vi "MSScript_SubVI_SentenceIdentifier.vi"(5 "IniPosition":i32, 6 "strlen":i32, 7 "Single sentance in":string) -> (0 "Delimiter SELs":cluster{"Start":u32, "End":u32}[](array[cluster]), 1 "Parameter string":cluster{"Str":string, "Start":i32}, 2 "Name string":cluster{"Str":string, "Start":i32}, 3 "Sentence type":string)   [LabVIEW 2018, in "MSScript.lvclass"]
uses:
  MSScript.lvclass
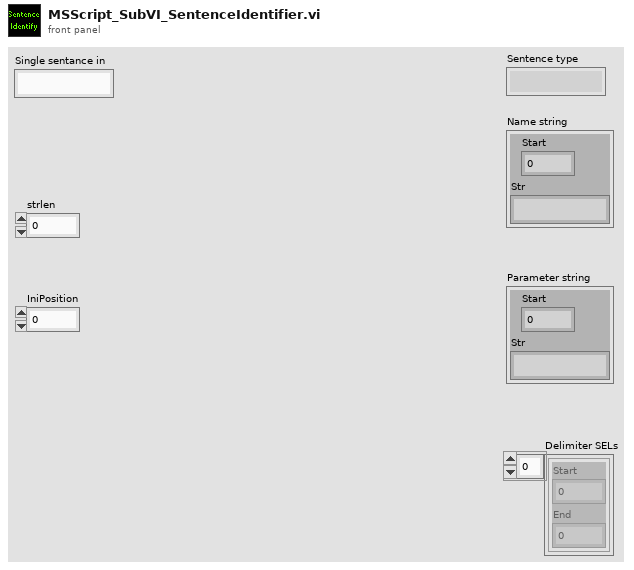
[diagram p1: front panel]
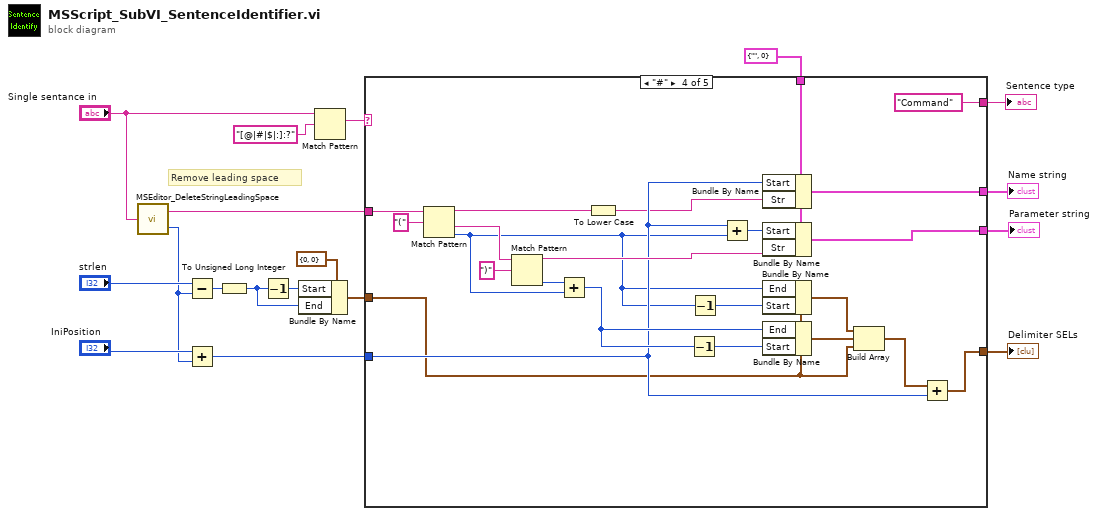
[diagram p0: block diagram]
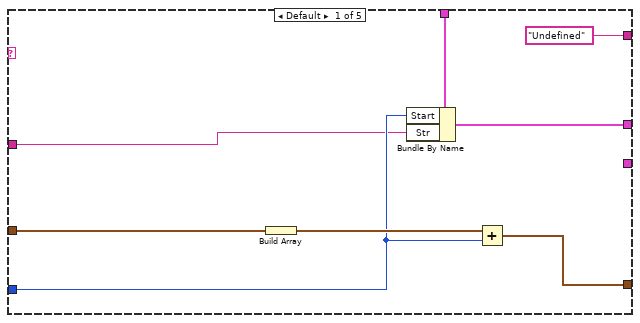
[diagram p2: hidden frame]
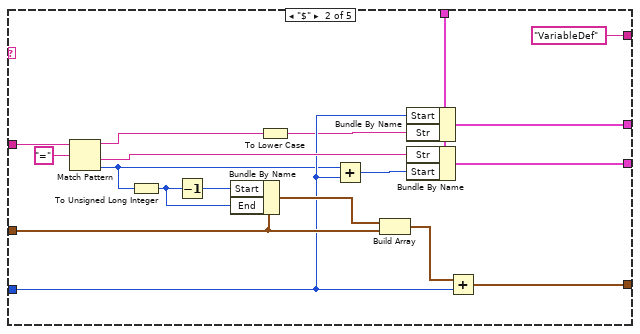
[diagram p3: hidden frame]
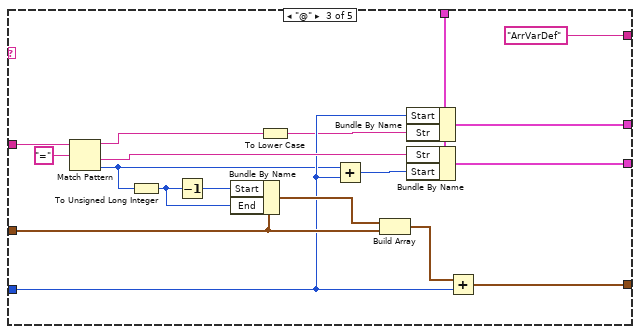
[diagram p4: hidden frame]
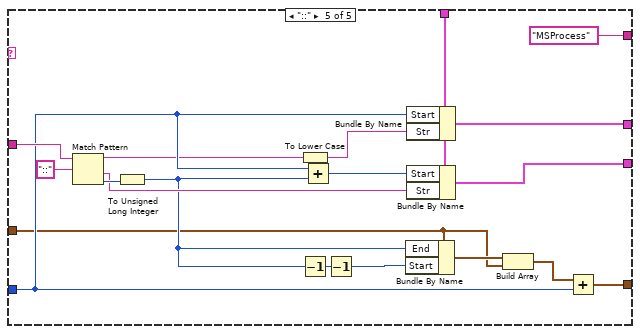
[diagram p5: hidden frame]
diagram:
  # "Remove leading space"
  n1 = call "MSEditor_DeleteStringLeadingSpace.vi"("string in"="Single sentance in") -> ("string after leading space"=w6:string, "offset past leading space"=w2:i32)
  n2 = Subtract(x="strlen", y=w2) -> (x-y=w4:i32)
  n3 = Add(x="IniPosition", y=w2) -> (x+y=w1:i32)
  n4 = To Unsigned Long Integer(number=w4) -> (unsigned 32bit integer=w10:u32)
  n5 = Decrement(x=w10) -> (x-1=w17:u32)
  n6 = Bundle By Name(cluster=cluster{"Start":u32, "End":u32} {"Start"=0, "End"=0}, "Start"=w17, "End"=w10) -> (w16:cluster{"Start":u32, "End":u32})
  n7 = Match Pattern(string="Single sentance in", regular expression="[@|#|$|:]:?") -> (match substring=w18:string)  [unwired: 1 in, 3 out]
  n8 = case shown="\"#\"" w18 {
    tunnel: w6 -> [w20 w35 w53 w81 w103]
    tunnel: ["Undefined" "VariableDef" "ArrVarDef" "Command" "MSProcess"] -> w14
    tunnel: w16 -> [w25 w38 w56 w65 w89]
    tunnel: [w23 w37 w55 w71 w95] -> w15
    tunnel: [_ w39 w57 w78 w102] -> w12
    tunnel: [w19 w29 w47 w80 w91] -> w13
    tunnel: cluster{"Str":string, "Start":i32} {"Str"="", "Start"=0} -> [w22 w30 w48 w67 w90]
    tunnel: w1 -> [w21 w33 w51 w69 w94]
    frame Default {
      n9 = Build Array(w25) -> (w24:cluster{"Start":u32, "End":u32}[])
      n10 = Bundle By Name(cluster=w22, "Start"=w21, "Str"=w20) -> (w19:cluster{"Str":string, "Start":i32})
      n11 = Add(x=w24, y=w21) -> (x+y=w23:cluster{"Start":u32, "End":u32}[])
    }
    frame "$" {
      n12 = Match Pattern(string=w35, regular expression="=") -> (before substring=w28:string, after substring=w34:string, offset past match=w32:i32)  [unwired: 1 in, 1 out]
      n13 = To Unsigned Long Integer(number=w32) -> (unsigned 32bit integer=w36:u32)
      n14 = Decrement(x=w36) -> (x-1=w42:u32)
      n15 = Bundle By Name(cluster=w38, "Start"=w42, "End"=w36) -> (w41:cluster{"Start":u32, "End":u32})
      n16 = To Lower Case(string=w28) -> (all lower case string=w27:string)
      n17 = Add(x=w32, y=w33) -> (x+y=w31:i32)
      n18 = Build Array(w41, w38) -> (w40:cluster{"Start":u32, "End":u32}[])
      n19 = Bundle By Name(cluster=w30, "Start"=w33, "Str"=w27) -> (w29:cluster{"Str":string, "Start":i32})
      n20 = Bundle By Name(cluster=w30, "Str"=w34, "Start"=w31) -> (w39:cluster{"Str":string, "Start":i32})
      n21 = Add(x=w40, y=w33) -> (x+y=w37:cluster{"Start":u32, "End":u32}[])
    }
    frame "@" {
      n22 = Match Pattern(string=w53, regular expression="=") -> (before substring=w46:string, after substring=w52:string, offset past match=w50:i32)  [unwired: 1 in, 1 out]
      n23 = To Unsigned Long Integer(number=w50) -> (unsigned 32bit integer=w54:u32)
      n24 = Decrement(x=w54) -> (x-1=w60:u32)
      n25 = Bundle By Name(cluster=w56, "Start"=w60, "End"=w54) -> (w59:cluster{"Start":u32, "End":u32})
      n26 = To Lower Case(string=w46) -> (all lower case string=w45:string)
      n27 = Add(x=w50, y=w51) -> (x+y=w49:i32)
      n28 = Build Array(w59, w56) -> (w58:cluster{"Start":u32, "End":u32}[])
      n29 = Bundle By Name(cluster=w48, "Start"=w51, "Str"=w45) -> (w47:cluster{"Str":string, "Start":i32})
      n30 = Bundle By Name(cluster=w48, "Str"=w52, "Start"=w49) -> (w57:cluster{"Str":string, "Start":i32})
      n31 = Add(x=w58, y=w51) -> (x+y=w55:cluster{"Start":u32, "End":u32}[])
    }
    frame "#" {
      n32 = Match Pattern(string=w81, regular expression="(") -> (before substring=w64:string, after substring=w82:string, offset past match=w68:i32)  [unwired: 1 in, 1 out]
      n33 = Match Pattern(string=w82, regular expression=")") -> (before substring=w79:string, offset past match=w77:i32)  [unwired: 1 in, 2 out]
      n34 = Add(x=w77, y=w68) -> (x+y=w75:i32)
      n35 = To Lower Case(string=w64) -> (all lower case string=w63:string)
      n36 = Decrement(x=w75) -> (x-1=w74:i32)
      n37 = Decrement(x=w68) -> (x-1=w76:i32)
      n38 = Add(x=w69, y=w68) -> (x+y=w70:i32)
      n39 = Bundle By Name(cluster=w67, "Start"=w69, "Str"=w63) -> (w80:cluster{"Str":string, "Start":i32})
      n40 = Bundle By Name(cluster=w67, "Start"=w70, "Str"=w79) -> (w78:cluster{"Str":string, "Start":i32})
      n41 = Bundle By Name(cluster=w65, "End"=w68, "Start"=w76) -> (w73:cluster{"Start":u32, "End":u32})
      n42 = Bundle By Name(cluster=w65, "End"=w75, "Start"=w74) -> (w66:cluster{"Start":u32, "End":u32})
      n43 = Build Array(w73, w66, w65) -> (w72:cluster{"Start":u32, "End":u32}[])
      n44 = Add(x=w72, y=w69) -> (x+y=w71:cluster{"Start":u32, "End":u32}[])
    }
    frame "::" {
      n45 = Match Pattern(string=w103, regular expression="::") -> (before substring=w88:string, after substring=w96:string, offset past match=w101:i32)  [unwired: 1 in, 1 out]
      n46 = To Unsigned Long Integer(number=w101) -> (unsigned 32bit integer=w93:u32)
      n47 = To Lower Case(string=w88) -> (all lower case string=w87:string)
      n48 = Decrement(x=w93) -> (x-1=w100:u32)
      n49 = Add(x=w94, y=w93) -> (x+y=w92:u32)
      n50 = Decrement(x=w100) -> (x-1=w86:u32)
      n51 = Bundle By Name(cluster=w89, "End"=w93, "Start"=w86) -> (w97:cluster{"Start":u32, "End":u32})
      n52 = Bundle By Name(cluster=w90, "Start"=w94, "Str"=w87) -> (w91:cluster{"Str":string, "Start":i32})
      n53 = Bundle By Name(cluster=w90, "Start"=w92, "Str"=w96) -> (w102:cluster{"Str":string, "Start":i32})
      n54 = Build Array(w97, w89) -> (w99:cluster{"Start":u32, "End":u32}[])
      n55 = Add(x=w99, y=w94) -> (x+y=w95:cluster{"Start":u32, "End":u32}[])
    }
  }
  "Delimiter SELs" <- w15
  "Sentence type" <- w14
  "Name string" <- w13
  "Parameter string" <- w12
